vi "Array Expressions and Generators.vi"() -> ()   [LabVIEW 2020, in "Examples.lvlib"]
doc: "Examples of using the array expression and generator VIs to generate arrays in a declarative manner."
uses:
  Examples.lvlib
  ca22692f-5589-4394-aacc-342ac0da72c5.vi
  5edb8a6f-6f4e-424e-819b-23cf34166abd.vi
  5dd71f54-0758-47bf-bba6-44a4c3450041.vi
  2182861f-b3fb-400c-b44d-44ce1d348bbe.vi
  ca22692f-5589-4394-aacc-342ac0da72c5.vi/35c0bed4-0107-49e5-a1be-c3402b1a4269.vi
  ca22692f-5589-4394-aacc-342ac0da72c5.vi/4b1c2d87-9503-4854-8dc7-31bb0771dd1b.vi
  5edb8a6f-6f4e-424e-819b-23cf34166abd.vi/35c0bed4-0107-49e5-a1be-c3402b1a4269.vi
  5edb8a6f-6f4e-424e-819b-23cf34166abd.vi/4b1c2d87-9503-4854-8dc7-31bb0771dd1b.vi
  5edb8a6f-6f4e-424e-819b-23cf34166abd.vi/4049b438-30ac-40ac-bf8b-38a25aeeaacb.vi
  5dd71f54-0758-47bf-bba6-44a4c3450041.vi/6603e637-5b00-4c85-831f-438498c6f5cd.vi
  5dd71f54-0758-47bf-bba6-44a4c3450041.vi/435e0bdd-08e9-4973-aa49-bb73efdc2477.vi
  <vilib>/dlg_ctls.llb/Space Constant.vi
  5dd71f54-0758-47bf-bba6-44a4c3450041.vi/b24c019a-0099-4d06-9010-75d0c3ff117b.vi
  2182861f-b3fb-400c-b44d-44ce1d348bbe.vi/6603e637-5b00-4c85-831f-438498c6f5cd.vi
  2182861f-b3fb-400c-b44d-44ce1d348bbe.vi/435e0bdd-08e9-4973-aa49-bb73efdc2477.vi
  2182861f-b3fb-400c-b44d-44ce1d348bbe.vi/48c7ac7e-bb0d-49e2-af2c-796dbdcbcaf5.vi
  5dd71f54-0758-47bf-bba6-44a4c3450041.vi/6603e637-5b00-4c85-831f-438498c6f5cd.vi/35c0bed4-0107-49e5-a1be-c3402b1a4269.vi
  5dd71f54-0758-47bf-bba6-44a4c3450041.vi/6603e637-5b00-4c85-831f-438498c6f5cd.vi/4b1c2d87-9503-4854-8dc7-31bb0771dd1b.vi
  5dd71f54-0758-47bf-bba6-44a4c3450041.vi/435e0bdd-08e9-4973-aa49-bb73efdc2477.vi/35c0bed4-0107-49e5-a1be-c3402b1a4269.vi
  5dd71f54-0758-47bf-bba6-44a4c3450041.vi/435e0bdd-08e9-4973-aa49-bb73efdc2477.vi/4b1c2d87-9503-4854-8dc7-31bb0771dd1b.vi
  5dd71f54-0758-47bf-bba6-44a4c3450041.vi/435e0bdd-08e9-4973-aa49-bb73efdc2477.vi/4049b438-30ac-40ac-bf8b-38a25aeeaacb.vi
  2182861f-b3fb-400c-b44d-44ce1d348bbe.vi/6603e637-5b00-4c85-831f-438498c6f5cd.vi/35c0bed4-0107-49e5-a1be-c3402b1a4269.vi
  2182861f-b3fb-400c-b44d-44ce1d348bbe.vi/6603e637-5b00-4c85-831f-438498c6f5cd.vi/4b1c2d87-9503-4854-8dc7-31bb0771dd1b.vi
  2182861f-b3fb-400c-b44d-44ce1d348bbe.vi/435e0bdd-08e9-4973-aa49-bb73efdc2477.vi/35c0bed4-0107-49e5-a1be-c3402b1a4269.vi
  2182861f-b3fb-400c-b44d-44ce1d348bbe.vi/435e0bdd-08e9-4973-aa49-bb73efdc2477.vi/4b1c2d87-9503-4854-8dc7-31bb0771dd1b.vi
  2182861f-b3fb-400c-b44d-44ce1d348bbe.vi/435e0bdd-08e9-4973-aa49-bb73efdc2477.vi/4049b438-30ac-40ac-bf8b-38a25aeeaacb.vi
panel:
  out "D":u16[](array[numeric])
  out "C":dbl[](array[numeric]) format="%.2f"
  out "B":i32[](array[numeric])
  out "A":dbl[](array[numeric]) format="%.2f"
  # "1) View the block diagram to inspect the various array expressions and generators.\n2) Run the VI and view the front panel to see the results."
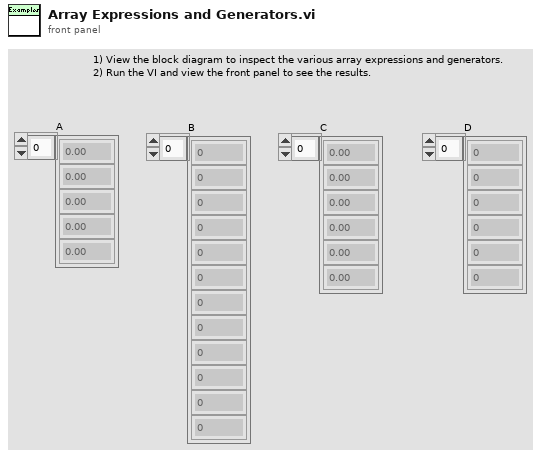
[diagram p1: front panel]
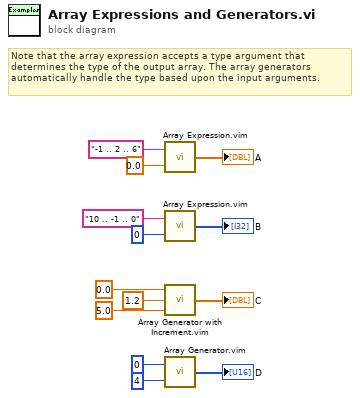
[diagram p0: block diagram]
diagram:
  # "Note that the array expression accepts a type argument that determines the type of the output array. The array generators automatically handle the type based upon the input arguments."
  n1 = call "Array Expression.vim"("Type"=0.0, "Expression"="-1 .. 2 .. 6") -> ("Array"=→"A":dbl[])
  n2 = call "Array Expression.vim"("Type"=0, "Expression"="10 .. -1 .. 0") -> ("Array"=→"B":i32[])
  n3 = call "Array Generator with Increment.vim"("Until"=5.0, "Increment"=1.2, "Begin"=0.0) -> ("Array"=→"C":dbl[])
  n4 = call "Array Generator.vim"("End"=u16 4, "Begin"=u16 0) -> ("Array"=→"D":u16[])
